vi "Run.vi"(8 "error in (no error)":errorcluster caption="entrée d'erreur (pas d'erreur)", 9 "y_pred":string[][](array[string]), 10 "y_true":string[][](array[string]), 11 "Mean_Gamma_Deviance.lvclass":refnum<class "Mean_Gamma_Deviance.lvclass">) -> (0 "error out":errorcluster caption="sortie d'erreur", 2 "String Data":string, 3 "Mean_Gamma_Deviance.lvclass":refnum<class "Mean_Gamma_Deviance.lvclass">)   [LabVIEW 2020, in "Mean_Gamma_Deviance.lvclass"]
doc: "Returns : \n\n- loss : float\nA non-negative floating point value (the best value is 0.0)."
uses:
  Mean_Gamma_Deviance.lvclass
  Mean_Gamma_Deviance.lvclass/Mean_Gamma_Deviance.ctl
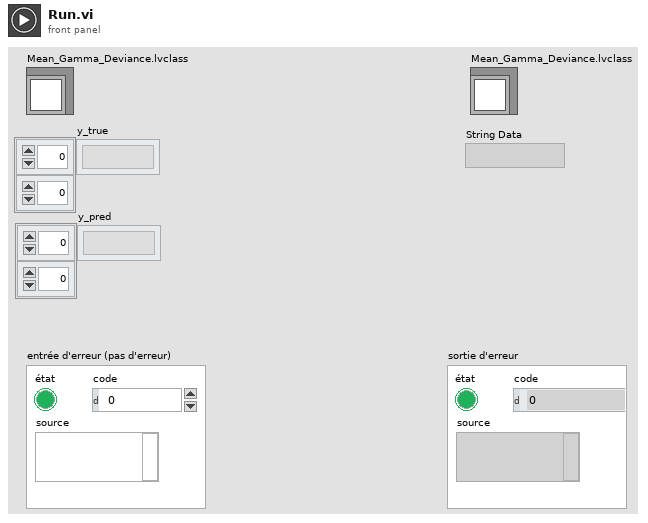
[diagram p1: front panel]
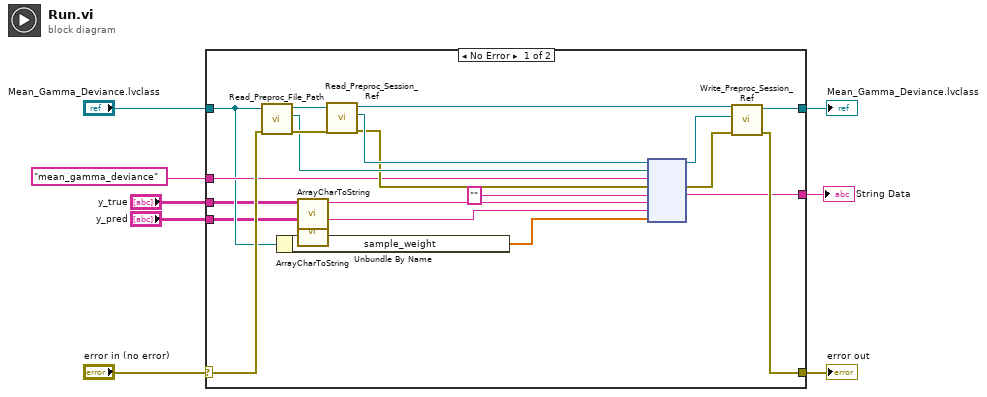
[diagram p0: block diagram]
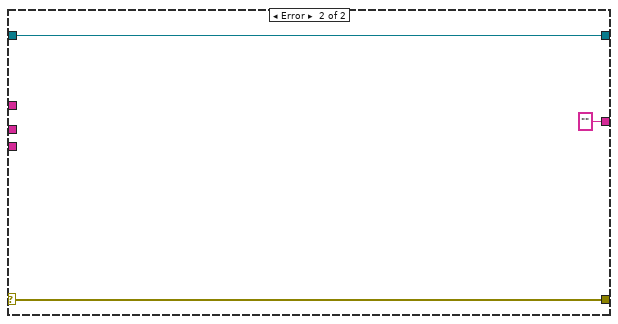
[diagram p2: hidden frame]
diagram:
  n1 = case shown="No Error" "error in (no error)" {
    selector: "error in (no error)" -> [w17 w31]
    tunnel: [w18 w31] -> w7
    tunnel: [w19 w30] -> w5
    tunnel: "Mean_Gamma_Deviance.lvclass" -> [w14 w30]
    tunnel: "mean_gamma_deviance" -> [w16 _]
    tunnel: [w15 ""] -> w4
    tunnel: "y_true" -> [w12 _]
    tunnel: "y_pred" -> [w11 _]
    frame No Error {
      n2 = call-dynamic "Read_Preproc_File_Path.vi"("error in (no error)"=w17, "Python in"=w14) -> ("error out"=w27:errorcluster, "File_Path"=w26:path, "Python out"=w28:refnum<class "Mean_Gamma_Deviance.lvclass">)  [unwired: 7 in]
      n3 = Unbundle By Name(w14) -> ("sample_weight"=w13:dbl[])
      n4 = call "ArrayCharToString.vi"("TAB"=w12) -> ("Instruction"=w10:string)  [unwired: 10 in]
      n5 = call "ArrayCharToString.vi"("TAB"=w11) -> ("Instruction"=w9:string)  [unwired: 10 in]
      n6 = call-dynamic "Read_Preproc_Session_Ref.vi"("error in (no error)"=w27, "Python in"=w28) -> ("error out"=w24:errorcluster, "Session_ref"=w25:refnum<k35>, "Python out"=w23:refnum<class "Mean_Gamma_Deviance.lvclass">)  [unwired: 7 in]
      n7 = node(w25, w26, w16, w24, "", w10, w9, w13) -> (w21:refnum<k35>, w22:errorcluster, w15:string)  [unwired: 3 in, 2 out]
      n8 = call-dynamic "Write_Preproc_Session_Ref.vi"("error in (no error)"=w22, "Session_ref"=w21, "Python in"=w23) -> ("error out"=w18:errorcluster, "Python out"=w19:refnum<class "Mean_Gamma_Deviance.lvclass">)  [unwired: 7 in]
    }
    frame Error {
    }
  }
  "error out" <- w7
  "Mean_Gamma_Deviance.lvclass" <- w5
  "String Data" <- w4
